vi "Tilt.vi"(11 "Array in":string[](array[string])) -> (3 "Array out":string[](array[string]))   [LabVIEW 2021]
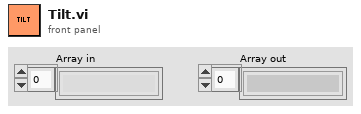
[diagram p1: front panel]
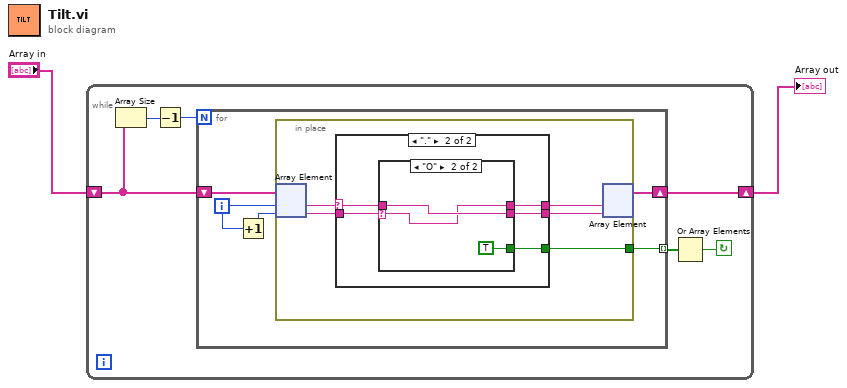
[diagram p0: block diagram]
diagram:
  n1 = while {
    shift-right: [w6] -> w2
    shift-left: "Array in" -> [w5]
    stop <- w3 continue-if-true
    n2 = Array Size(array=w5) -> (size(s)=w8:i32)
    n3 = Decrement(x=w8) -> (x-1=w7:i32)
    n4 = for {
      N: w7 -> [_]
      shift-right: [w12] -> w6
      shift-left: w5 -> [w13]
      tunnel: [w9] -> w4 mode=indexing
      i -> [w10]
      n5 = Increment(x=w10) -> (x+1=w11:i32)
      n6 = in-place {
        in-place-border: [w14] -> w9
        n7 = in-place-array #1(w13, w10, w11) -> (w18:string, w17:string)
        n8 = case shown="\".\"" w18 {
          selector: w18 -> [w20 w23]
          tunnel: w17 -> [w19 w25]
          tunnel: [w20 w24] -> w16
          tunnel: [w19 w22] -> w15
          tunnel: [_ w21] -> w14
          frame Default {
          }
          frame "." {
            n9 = case shown="\"O\"" w25 {
              selector: w25 -> [w26 w29]
              tunnel: [w27 w29] -> w24
              tunnel: w23 -> [w27 w30]
              tunnel: [w26 w30] -> w22
              tunnel: [_ TRUE] -> w21
              frame Default {
              }
              frame "O" {
              }
            }
          }
        }
        n10 = in-place-array #1(w16, w15) -> (w12:string[])  [unwired: 2 out]
      }
    }
    n11 = Or Array Elements(Boolean array=w4) -> (logical OR=w3:bool)
  }
  "Array out" <- w2
